vi "Acq Configure Channel.vi"(0 "session in":refnum<class "Digitizer Control.lvclass">, 1 "desired AI range (V)":dbl[](array[numeric]), 2 "desired AI offset (V)":dbl[](array[numeric]), 4 "sampling rate (SPS)":dbl, 5 "error in (no error)":errorcluster, 6 "AI channel":string) -> (11 "sample scale factor":dbl[](array[numeric]), 13 "DSP delay (s)":dbl, 14 "session out":refnum<class "Digitizer Control.lvclass">, 15 "actual AI range (V)":dbl[](array[numeric]), 16 "actual AI offset (V)":dbl[](array[numeric]), 18 "actual sampling rate (SPS)":dbl, 19 "error out":errorcluster)   [LabVIEW 2021, in "Digitizer Control.lvclass"]
doc: "Configures the acquisition channel parameters, such as the input channel and the sampling rate. Use the <B>Acq Configure Start Trigger.vi</B> to configure the start trigger, and the <B>Acq Configure Transfer.vi</B> to configure the waveform transfer. Once the acquisition is configured, use the <B>Acq Initiate.vi</B> to initiate an acquisition, then use the <B>Acq Fetch Waveform.vi</B> to fetch the acquired samples. Use the <B>Acq Get Status.vi</B> to check the acquisition status and the <B>Acq Stop.vi</B> to stop an acquisition.\n\nInputs:\n\n<B>session in</B>: The device session.\n\n<B>AI channel</B>: The AI channel(s) to enable, this input can be \"AI0\", \"AI1\" or \"AI0,AI1\". NOTE: changing the enabled channels invalidates the transfer configuration in which case the <B>Acq Configure Transfer.vi</B> should be called (again) to reconfigure the transfer.\n\n<B>AI range (V)</B>: The desired vertical range of the channels, given in Volts. This input is an array, the n-th element corresponds to the n-th channel.\n\n<B>AI offset (V)</B>: The desired vertical offset of the channels, given in Volts. This input is an array, the n-th element corresponds to the n-th channel.\n\n<B>sampling rate</B>: The desired sampling rate, in SPS, of the acquired waveform.\n\nOutputs:\n\n<B>session out</B>: The device session passed on the <B>session in</B> input.\n\n<B>actual AI range (V)</B>: The actual vertical range of the channels, given in Volts. This output is an array, the n-th element corresponds to the n-th channel.\n\n<B>actual AI offset (V)</B>: The actual vertical offset of the channels, given in Volts. This output is an array, the n-th element corresponds to the n-th channel.\n\n<B>actual sampling rate</B>: The actual sampling rate, in SPS, used by the acquisition.\n\n<B>DSP delay (s)</B>: The minimum delay the acquisition DSP path supports using the current configuration.\n\n<B>sample scale factor</B>: Scale factor for converting between Voltage levels and the numbers transferred by the FPGA Target. Multiply the integer samples returned by the FPGA Target by <B>sample scale factor</B> * 2^-(<B>sample size (bits)</B>) to obtain Voltage levels. NOTE: <B>sample size (bits)</B> is an output of the <B>Acq Configure Transfer.vi</B>."
uses:
  Digitizer Control.lvclass
  Digitizer Control.lvclass/Digitizer Control.ctl
  <vilib>/Utility/error.llb/Error Cluster From Error Code.vi
  <vilib>/rvi/errors/niLvFpgaAdjustHostInterfaceError.vi
  <instrlib>/FlexRIO/API/Host/v1/NI FlexRIO/API/Get Property Reference - Fpga Small.vi
  <vilib>/rvi/interface/nirviReadWriteControl/nirviReadWriteControl.xnode
  <resource>/objmgr/niflexrioapiChannel.rc
  <instrlib>/FlexRIO/API/Host/v1/NI FlexRIO API v1.lvlib
  <resource>/objmgr/niflexrioapi.rc
  <vilib>/rvi/interface/Simulation/niFpgaSimulationCallBeginRW.vi
  <instrlib>/_niInstr/Streaming/v1/Host/niInstr Streaming v1 Host.lvlib
  NiFpgaLv.dll
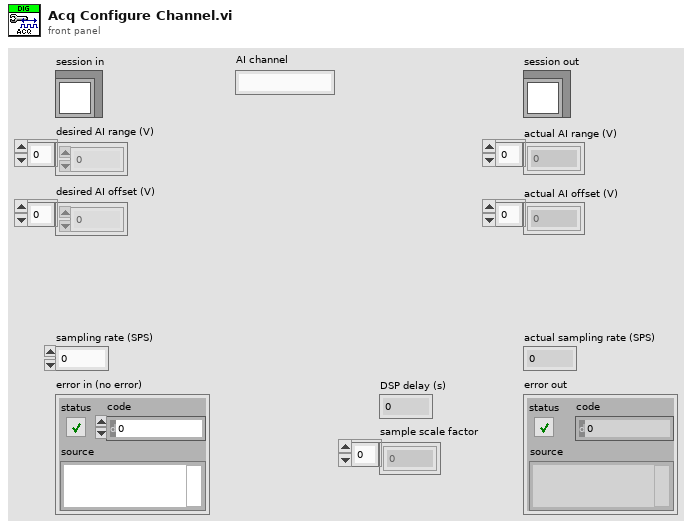
[diagram p1: front panel]
types:
  T1 = typedef "Digitizer Control.lvclass/Acq Session Data.ctl" = cluster{"ADC sampling rate":dbl, "SCTL rate":dbl, "DMA element size (bits)":i32, "sample size (bits)":i32[], "DMA/memory interface width (DMA elements)":i32, "transfer size (bits)":i32[], "stream instance":i32[], "trigger instance":u32, "group delay (s)":dbl, "data delay (s)":dbl, "target delay (s)":dbl, "trigger tracking enabled":bool, "channel configured":bool, "enabled channels":bool[], "transfer configured":bool, "dsp bypass":bool, "fractional decimator input rate":dbl, "fractional decimator output rate":dbl, "sample scale factor":dbl[], "memory size":u64[], "FIFO size":u64}
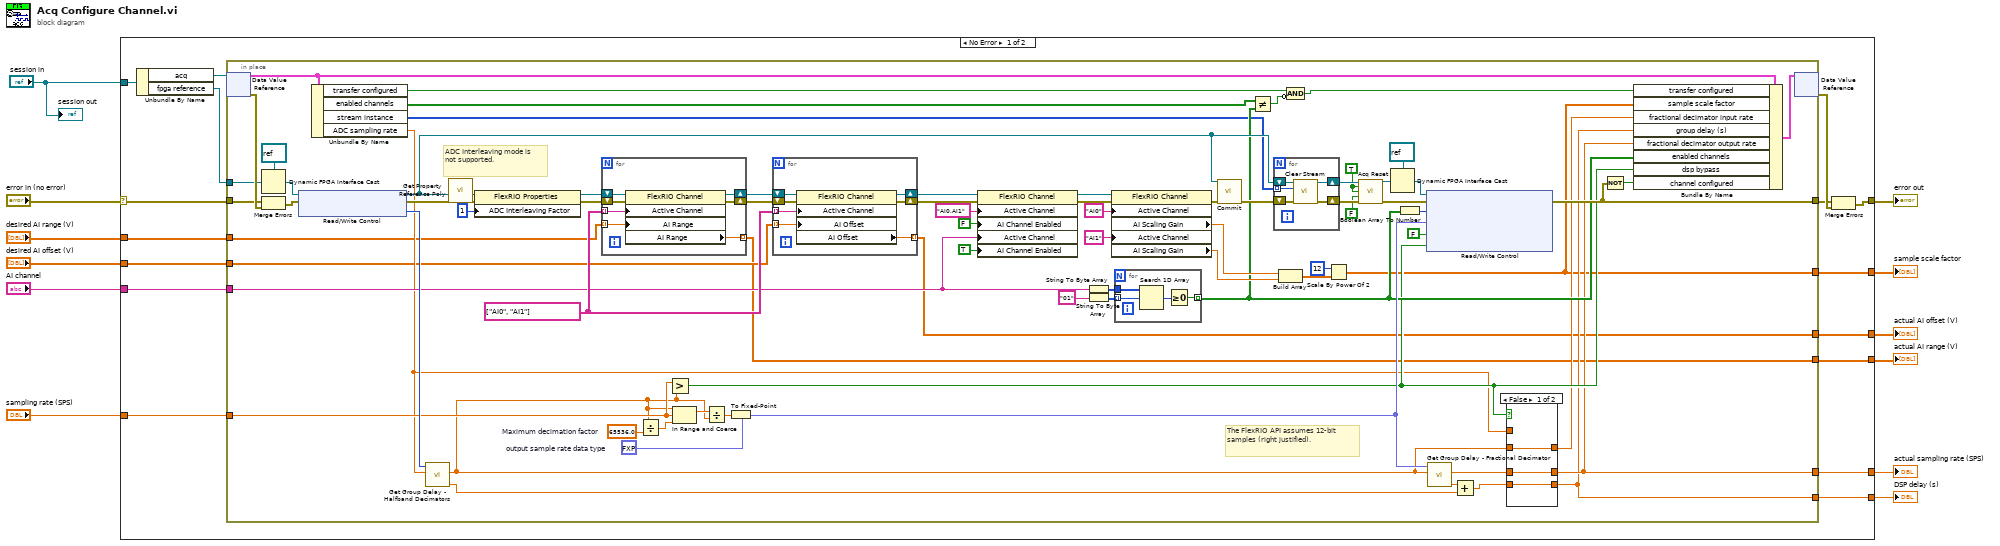
[diagram p0: block diagram]
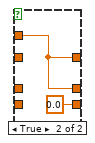
[diagram p2: hidden frame]
diagram:
  n1 = case shown="No Error" "error in (no error)" {
    selector: "error in (no error)" -> [w24 w135]
    tunnel: "AI channel" -> [w25 _]
    tunnel: "sampling rate (SPS)" -> [w27 _]
    tunnel: [w26 _] -> w9
    tunnel: "session in" -> [w20 _]
    tunnel: [w21 w135] -> w8
    tunnel: [w23 _] -> w7
    tunnel: [w17 _] -> w5
    tunnel: "desired AI range (V)" -> [w16 _]
    tunnel: "desired AI offset (V)" -> [w15 _]
    tunnel: [w14 _] -> w1
    tunnel: [w13 _] -> w2
    frame No Error {
      n2 = Unbundle By Name(w20) -> ("acq"=w19:refnum<data-value>, "fpga reference"=w18:refnum<k20>)
      n3 = in-place {
        in-place-border: w27 -> [w48]
        in-place-border: [w44] -> w26
        in-place-border: w25 -> [w70]
        in-place-border: [w105] -> w22
        in-place-border: w24 -> [w82]
        in-place-border: [w42] -> w23
        in-place-border: w18 -> [w68]
        in-place-border: [w39] -> w17
        in-place-border: w16 -> [w36]
        in-place-border: w15 -> [w33]
        in-place-border: [w30] -> w14
        in-place-border: [w29] -> w13
        w106 = string[] ["AI0", "AI1"]
        w66 = TRUE
        w93 = fxp<+,48,1> 0.0  # output sample rate data type
        w96 = 65536.0  # Maximum decimation factor
        # "ADC Interleaving mode is not supported."
        # "The FlexRIO API assumes 12-bit samples (right justified)."
        n4 = in-place-dvr #1(w19) -> (w102:T1, w100:errorcluster)
        n5 = Merge Errors(w82, w100) -> (w101:errorcluster)
        n6 = Dynamic FPGA Interface Cast(Session In=refnum<k20> refnum ("FPGA Interface"), Type=w68) -> (Session Out=w83:refnum<k20>)
        n7 = xnode "Read/Write Control"("FPGA VI Reference In"=w83, "error in"=w101) -> ("FPGA VI Reference Out"=w103:refnum<k20>, "error out"=w104:errorcluster, "acq.dsp.hb decimators"=w81:u8)
        n8 = Unbundle By Name(w102) -> ("transfer configured"=w50:bool, "enabled channels"=w53:bool[], "stream instance"=w52:i32[], "ADC sampling rate"=w41:dbl)
        n9 = call "Get Group Delay - Halfband Decimators.vi"("sampling rate in"=w41, "# of hb decimators"=w81) -> ("group delay (s)"=w61:dbl, "sampling rate out"=w40:dbl)  [unwired: 8 in]
        n10 = call-poly <instrlib>:"Get Property Reference Poly.vi"("error in (no error)"=w104, "fpga interface in"=w103) -> ("error out"=w86:errorcluster, "property reference"=w85:refnum<k20>)  [unwired: 4 in, 1 out]
        n11 = property class="FlexRIO Properties"(reference=w85, error in=w86, "ADC Interleaving Factor"=1 ("Device:ADC:Interleaving Factor")) -> (reference out=w37:refnum<k20>, error out=w38:errorcluster)
        n12 = for {
          shift-right: [w116] -> w35
          shift-left: w38 -> [w119]
          shift-right: [w120] -> w34
          shift-left: w37 -> [w118]
          tunnel: w36 -> [w117] mode=indexing
          tunnel: w106 -> [w115] mode=indexing
          tunnel: [w114] -> w29 mode=indexing
          n13 = property class="FlexRIO Channel"(reference=w118, error in=w119, "Active Channel"=w115, "AI Range"=w117) -> (reference out=w120:refnum<k20>, error out=w116:errorcluster, "AI Range"=w114:dbl)
        }
        n14 = Divide(x=w40, y=w96) -> (x/y=w97:dbl)
        n15 = Greater?(x=w48, y=w40) -> (0:w47:bool)
        n16 = In Range and Coerce(upper limit=w40, x=w48, lower limit=w97) -> (coerced(x)=w95:dbl)  [unwired: 1 out]
        n17 = Divide(x=w95, y=w40) -> (x/y=w94:dbl)
        n18 = To Fixed-Point(fixed-point type=w93, number=w94) -> (fixed-point=w79:fxp<+,48,1>)
        n19 = for {
          shift-right: [w109] -> w32
          shift-left: w35 -> [w112]
          shift-right: [w113] -> w31
          shift-left: w34 -> [w111]
          tunnel: w33 -> [w110] mode=indexing
          tunnel: w106 -> [w108] mode=indexing
          tunnel: [w107] -> w30 mode=indexing
          n20 = property class="FlexRIO Channel"(reference=w111, error in=w112, "Active Channel"=w108, "AI Offset"=w110) -> (reference out=w113:refnum<k20>, error out=w109:errorcluster, "AI Offset"=w107:dbl)
        }
        n21 = property class="FlexRIO Channel"(reference=w31, error in=w32, "Active Channel"="AI0,AI1", "AI Channel Enabled"=FALSE ("Analog Input:Enabled"), "Active Channel"=w70, "AI Channel Enabled"=TRUE ("Analog Input:Enabled")) -> (reference out=w71:refnum<k20>, error out=w72:errorcluster)
        n22 = String To Byte Array(string=w70) -> (unsigned byte array=w89:u8[])
        n23 = String To Byte Array(string="01") -> (unsigned byte array=w87:u8[])
        n24 = property class="FlexRIO Channel"(reference=w71, error in=w72, "Active Channel"="AI0", "Active Channel"="AI1") -> (error out=w62:errorcluster, "AI Scaling Gain"=w58:dbl, "AI Scaling Gain"=w57:dbl)  [unwired: 1 out]
        n25 = for {
          tunnel: w89 -> [w134]
          tunnel: w87 -> [w133] mode=indexing
          tunnel: [w131] -> w54 mode=indexing
          n26 = Search 1D Array(1D array=w134, element=w133) -> (index of element=w132:i32)  [unwired: 1 in]
          n27 = Greater Or Equal To 0?(x=w132) -> (x >= 0?=w131:bool)
        }
        n28 = call <instrlib>:"Commit.vi"("fpga interface in"=w103, "error in"=w62) -> ("error out"=w59:errorcluster)  [unwired: 12 in, 1 out]
        n29 = Not Equal?(x=w53, y=w54) -> (x != y?=w51:bool)
        n30 = for {
          tunnel: w52 -> [w127] mode=indexing
          shift-right: [w128] -> w75
          shift-left: w103 -> [w130]
          shift-right: [w129] -> w76
          shift-left: w59 -> [w126]
          n31 = call <instrlib>:"Clear Stream.vi"("error in (no error)"=w126, "stream index"=w127, "refnum in"=w130) -> ("error out"=w129:errorcluster, "refnum out"=w128:refnum<k20>)  [unwired: 7 in]
        }
        n32 = Build Array(w58, w57) -> (w56:dbl[])
        n33 = Compound Arithmetic op=AND(w50, invert w51) -> (w49:bool)
        n34 = Scale By Power Of 2(n=i16 12, x=w56) -> (x*2^n=w39:dbl[])
        n35 = call "Acq Reset.vi"("fpga reference in"=w75, "reset dsp"=w66, "reset stream control"=w66, "reset waveform streaming"=FALSE ("reset stream control"), "error in (no error)"=w76) -> ("fpga reference out"=w64:refnum<k20>, "error out"=w65:errorcluster)  [unwired: 9 in]
        n36 = Dynamic FPGA Interface Cast(Session In=refnum<k20> refnum ("FPGA Interface"), Type=w64) -> (Session Out=w98:refnum<k20>)
        n37 = Boolean Array To Number(Boolean array=w54) -> (number=w69:u32)
        n38 = xnode "Read/Write Control"("FPGA VI Reference In"=w98, "error in"=w65, "acq.channels enabled"=w69, "acq.dsp.output sample rate"=w79, "acq.stream.start enable"=FALSE, "acq.dsp.bypass"=w47) -> ("error out"=w105:errorcluster)  [unwired: 1 out]
        n39 = call "Get Group Delay - Fractional Decimator.vi"("sampling rate in"=w40, "output sample rate"=w79) -> ("group delay (s)"=w80:dbl, "sampling rate out"=w45:dbl)  [unwired: 8 in]
        n40 = Add(x=w80, y=w61) -> (x+y=w43:dbl)
        n41 = case shown="False" w47 {
          tunnel: w40 -> [w123 _]
          tunnel: [w123 w125] -> w46
          tunnel: w45 -> [w122 _]
          tunnel: [w122 w125] -> w44
          tunnel: w43 -> [w121 _]
          tunnel: [w121 0.0] -> w42
          tunnel: w41 -> [_ w125]
          frame False {
          }
          frame True {
          }
        }
        n42 = Not(x=w105) -> (.not. x?=w77:bool)
        n43 = Bundle By Name(cluster=w102, "transfer configured"=w49, "sample scale factor"=w39, "fractional decimator input rate"=w46, "group delay (s)"=w42, "fractional decimator output rate"=w44, "enabled channels"=w54, "dsp bypass"=w47, "channel configured"=w77) -> (w78:T1)
        n44 = in-place-dvr #1(w78) -> (w28:errorcluster)  [unwired: 1 out]
      }
      n45 = Merge Errors(w22, w28) -> (w21:errorcluster)
    }
    frame Error {
    }
  }
  "actual sampling rate (SPS)" <- w9
  "error out" <- w8
  "DSP delay (s)" <- w7
  "sample scale factor" <- w5
  "actual AI range (V)" <- w2
  "actual AI offset (V)" <- w1
  "session out" <- "session in"
